vi "UI-电源尾反面标签2检测.vi"(8 "error in (no error)":errorcluster caption="错误输入（无错误）", 11 "名称或相对路径":string="Template Program") -> (0 "error in (no error) 2":errorcluster caption="错误输入（无错误）")   [LabVIEW 2017]
uses:
  Global System.vi
  <vilib>/Utility/xml.llb/Write to XML File(string).vi
  Picture/SaveButtom.ctl
panel:
  in  "获取图像":bool
  in  "ROI获取":bool
  in  "创建模板":bool
  in  "保存图像":bool
  out "添加的路径":path
  in  "刷新":bool
  in  "测试按钮":bool
  in  "保存按钮":bool
  in  "Main":enum32{"主参数", "模板匹配参数 ", "测试效果"}(tab)
  in  "UI电源尾反面标签2基础参数":T1={"IsNorImage"=TRUE, "Exposure Values"=100289, "ImagePath"=path "C:/Users/hedongpo/Desktop/514-hdp/Alignment Assemble System/Test Picture/B/3.bmp"} caption="参数界面" {"Exposure Values" scale=0.0..200000.0}
  in  "UI电源尾反面标签2参数":T3={"Rectangle"={"Left"=0, "Top"=0, "Right"=0, "Bottom"=0, "Rotation"=0.0}, "Algorithm "=2, "Parameters"={"Number of Matches Requested"=1, "Minimum Match Score"=800.0, "Angle Ranges"=[{"Start Angle"=-180.0, "End Angle"=180.0}]}, "Advanced Options "=[{"Item"=102, "Value"=10.0}, {"Item"=106, "Value"=300.0}, {"Item"=107, "Value"=0.0}, {"Item"=108, "Value"=6.0}, {"Item"=109, "Value"=1.0}, {"Item"=114, "Value"=25.0}, {"Item"=111, "Value"=20.0}, {"Item"=112, "Value"=10.0}, {"Item"=113, "Value"=20.0}, {"Item"=103, "Value"=1.0}, {"Item"=104, "Value"=20.0}, {"Item"=105, "Value"=0.0}, {"Item"=100, "Value"=5.0}], "模板路径"=path "", "Color Plane "=0} {"Color Plane" items=["Red", "Green", "Blue", "Hue", "Saturation", "Luminance", "Value", "Intensity"]; "Advanced Options"."Item" items=["LD Sampling - Minimum Constrast"=0, "LD Sampling - Enable Subpixel Accuracy"=1, "LD Sampling - Search Strategy"=2, "LD Sampling - Subpixel Iterations"=3, "LD Sampling - Subpixel Tolerance"=4, "LD Sampling - Initial Match List Length"=5, "LD Sampling - Match List Reduction Factor"=6, "LD Sampling - Initial Step Size"=7, "LD Sampling - Intermediate Angular Accuracy"=8, "-"=9, "Pyramid - Max Pyramid Level"=100, "Pyramid - Minimum Contrast"=102, "Pyramid - Enable Subpixel Accuracy"=103, "Pyramid - Subpixel Iterations"=104, "Pyramid - Subpixel Tolerance"=105, "Pyramid - Initial Match List Length"=106, "Pyramid - Match List Reduction Factor"=107, "Pyramid - Intermediate Angular Accuracy"=108, "Pyramid - Process Border Matches"=109, "Pyramid - Min Match Separation Distance"=111, "Pyramid - Min Match Separation Angle"=112, "Pyramid - Max Match Overlap"=113, "Pyramid - Max Cache in MB"=114, "Pyramid - Clear Cache"=115, "-"=116, "Enable Defect Map"=200]; "Algorithm" items=["All", "Low Discrepancy Sampling", "Grayscale Value Pyramid", "Gradients Pyramid"]; "Rectangle"."Rotation" format="%.2f"; "Rectangle"."Left" scale=0.0..1024.0; "Rectangle"."Right" scale=0.0..1024.0}
  out "结果":bool
  out "原始图像":T4(plugin-control)
  out "模板图片":T4(plugin-control)
  out "路径输出":path
  in  "Vision Paramter Save Buttom":T5
  out "system time":string
  in  "取消按钮":bool
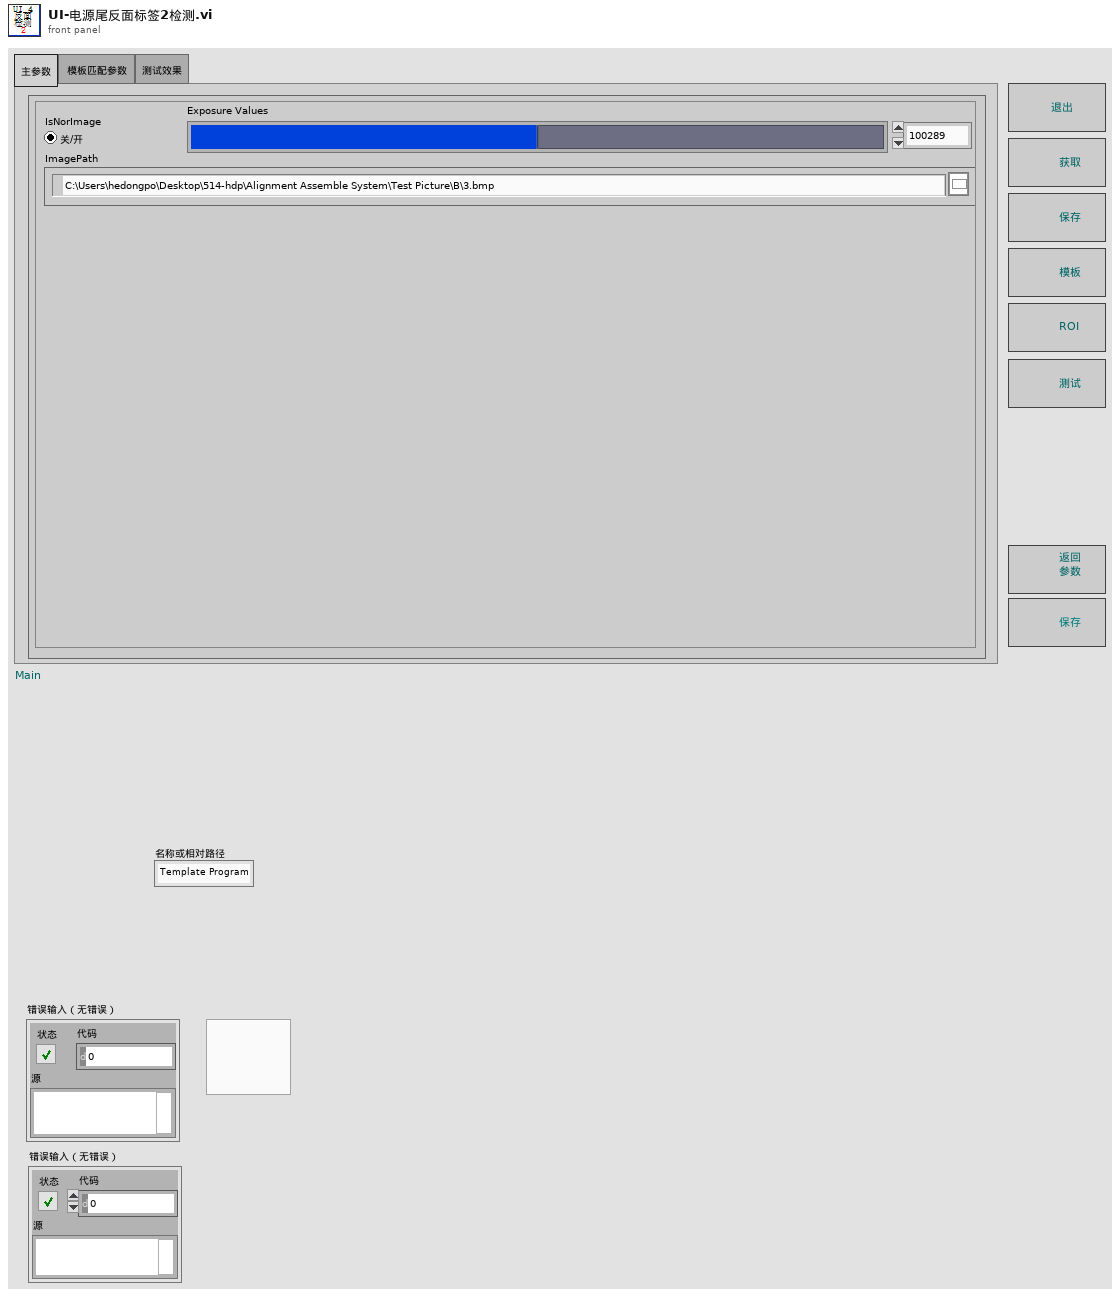
[diagram p1: front panel]
types:
  T1 = cluster{"IsNorImage":bool, "Exposure Values":u32, "ImagePath":path}
  T2 = typedef "IMAQ Rectangle" = cluster{"Left":i32, "Top":i32, "Right":i32, "Bottom":i32, "Rotation":dbl}
  T3 = cluster{"Rectangle":T2, "Algorithm ":i32, "Parameters":cluster{"Number of Matches Requested":i32, "Minimum Match Score":sgl, "Angle Ranges":cluster{"Start Angle":sgl, "End Angle":sgl}[]}, "Advanced Options ":cluster{"Item":u16, "Value":dbl}[], "模板路径":path, "Color Plane ":i32}
  T4 = typedef "IMAQ Image.ctl" = refnum<image>
  T5 = typedef "SaveButtom.ctl" = bool
  T6 = cluster{"index":i32, "this vi":refnum<vi>, "error out":errorcluster}
  T7 = cluster{"master data":string, "priority":u16, "secondary data":string[]}
  T8 = cluster{"case name":string[], "queue array":refnum<queue>[]}
  T9 = typedef "Image Type" = u32
  T10 = cluster{"Global Rectangle":i32[], "Contours":cluster{"Contour Type":u32, "ROI Type":u32, "Points":i32[]}[]}
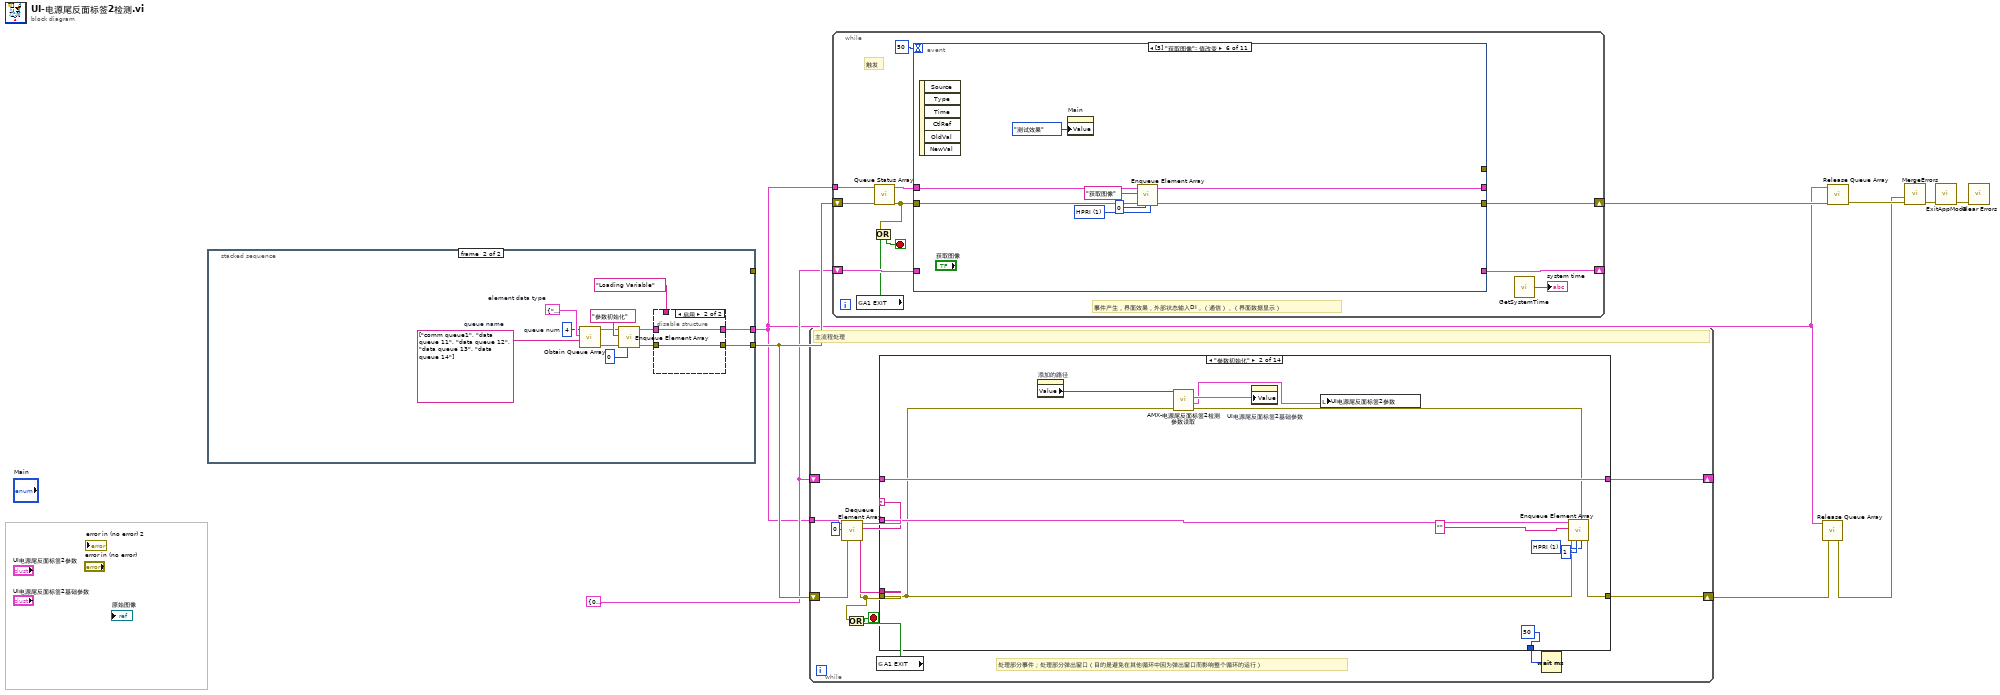
[diagram p0: block diagram]
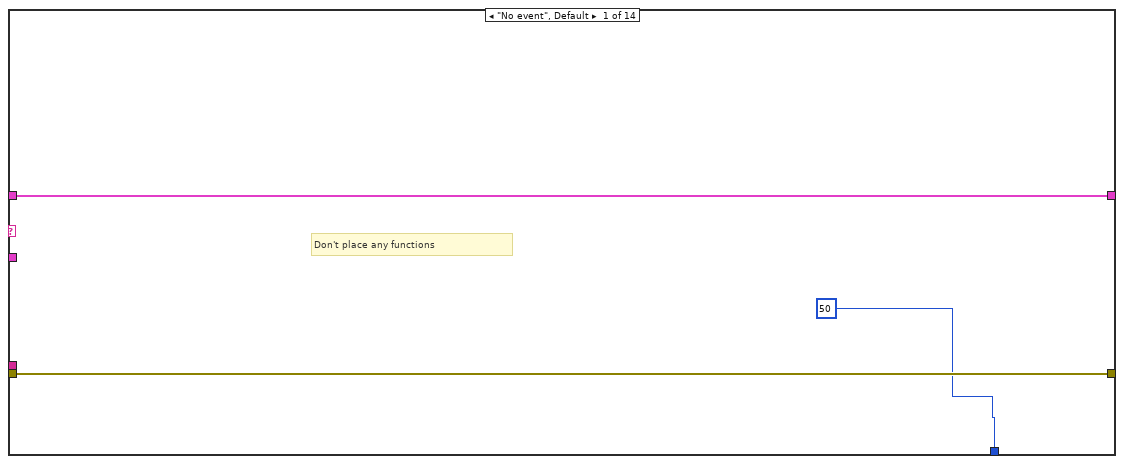
[diagram p2: hidden frame]
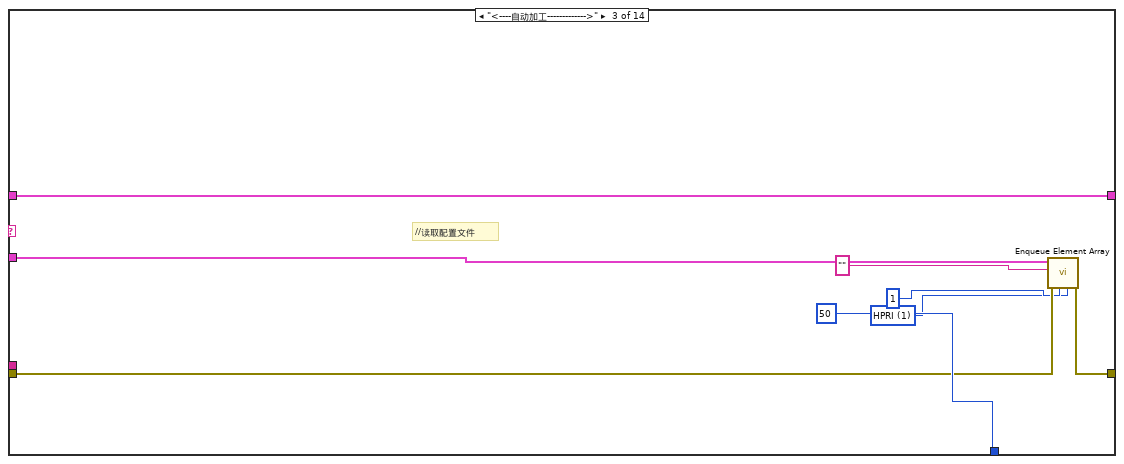
[diagram p3: hidden frame]
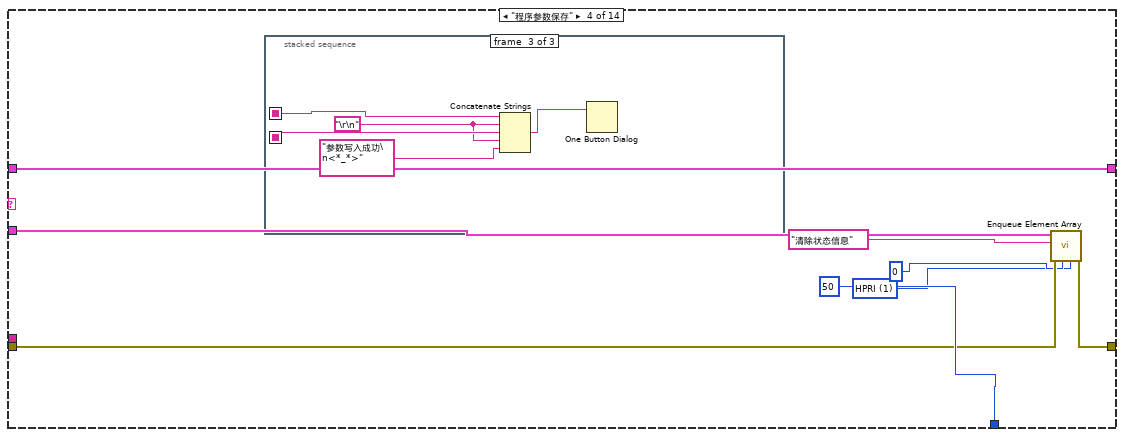
[diagram p4: hidden frame]
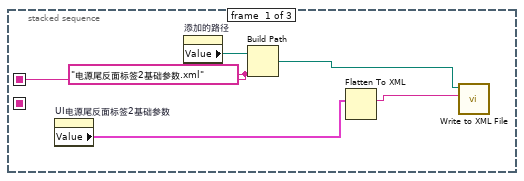
[diagram p5: hidden frame]
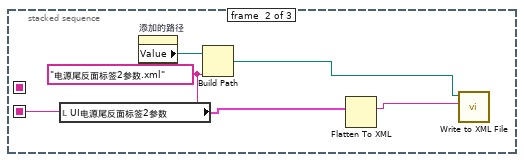
[diagram p6: hidden frame]
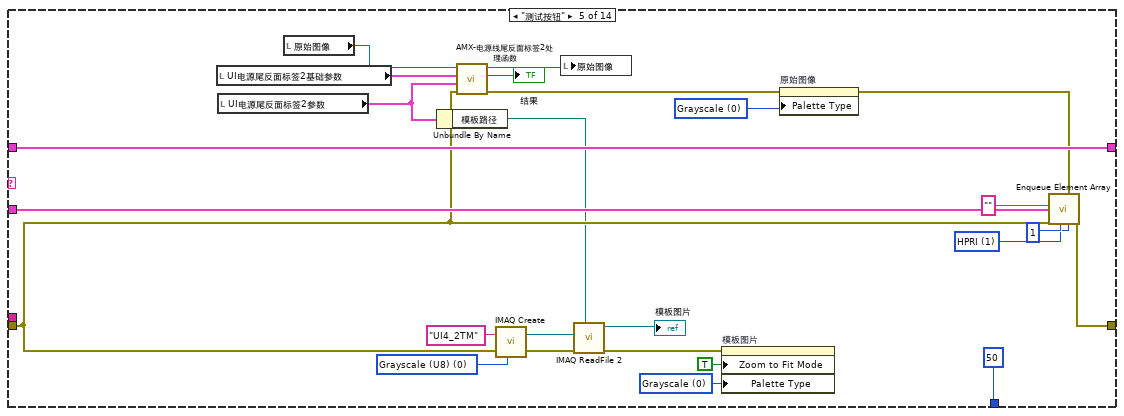
[diagram p7: hidden frame]
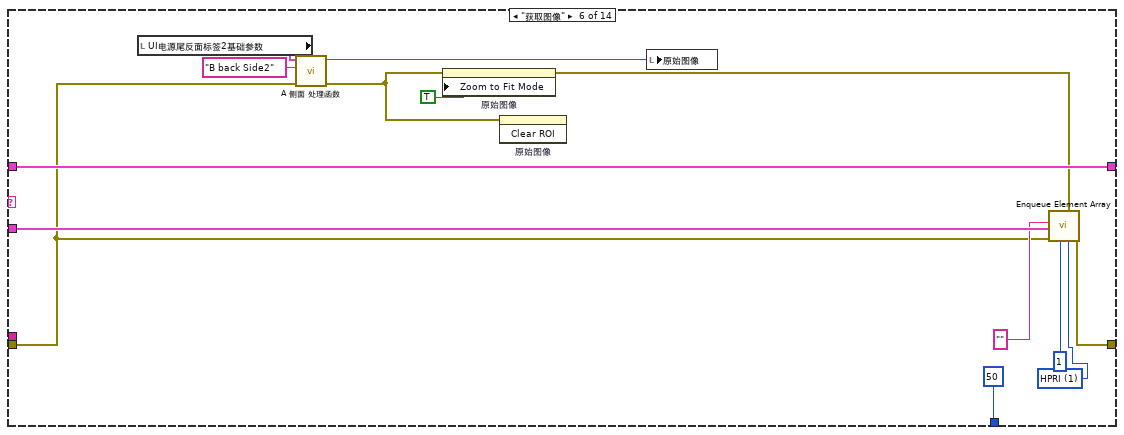
[diagram p8: hidden frame]
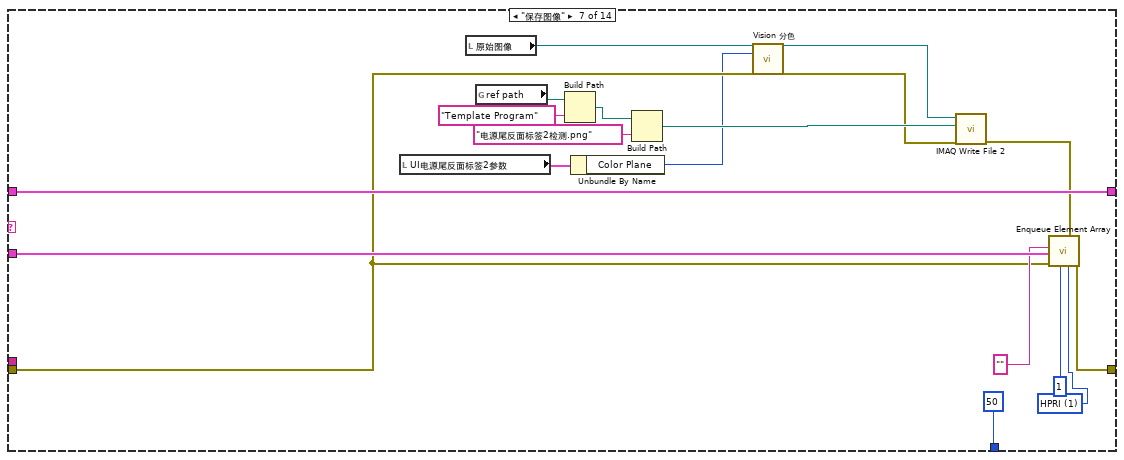
[diagram p9: hidden frame]
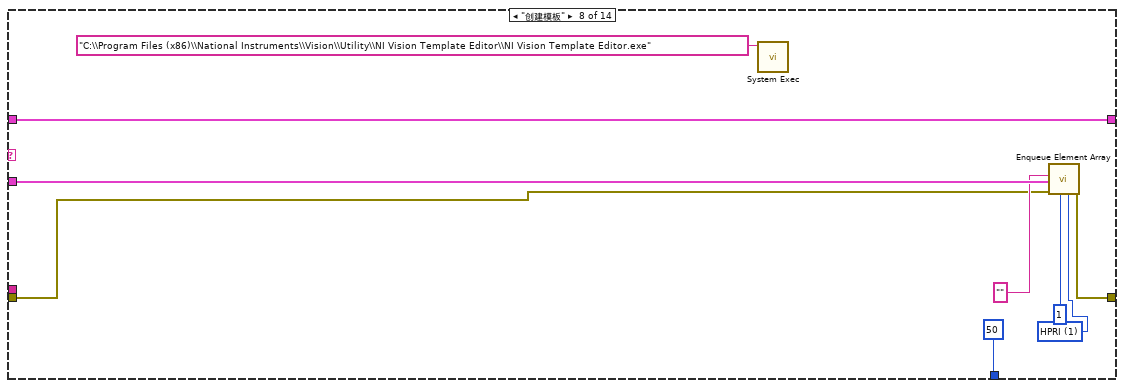
[diagram p10: hidden frame]
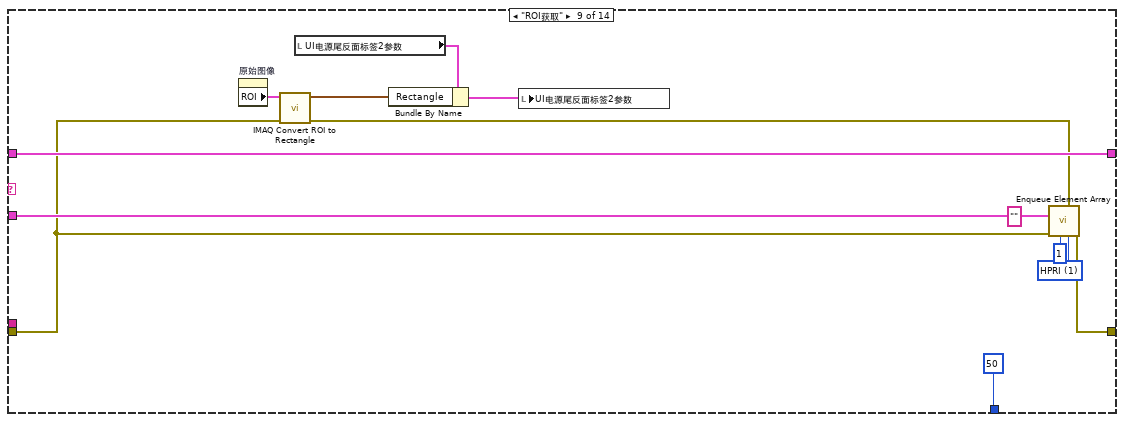
[diagram p11: hidden frame]
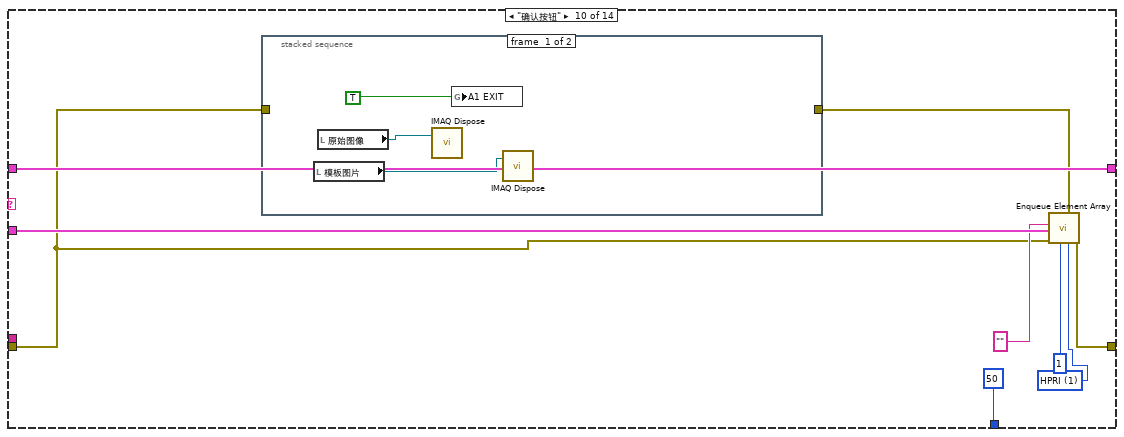
[diagram p12: hidden frame]
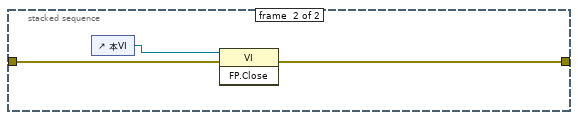
[diagram p13: hidden frame]
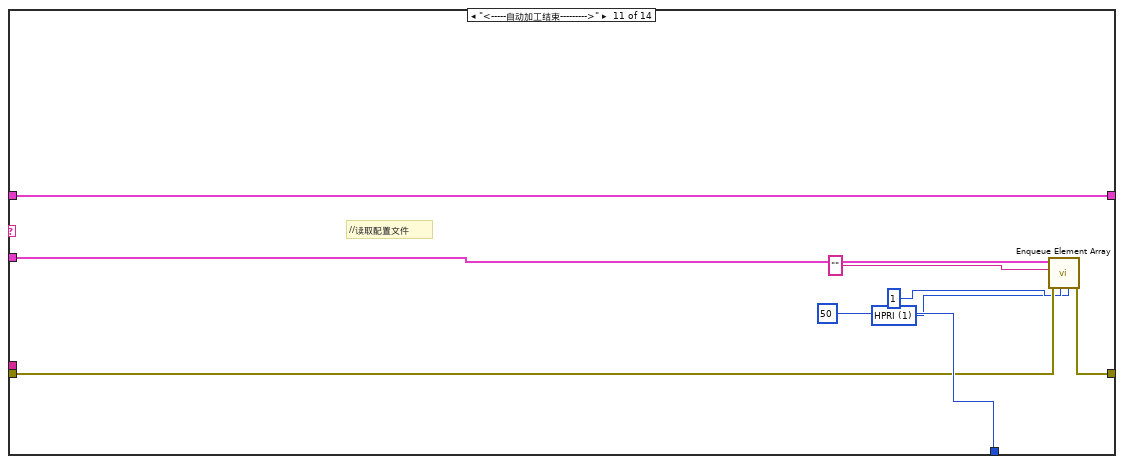
[diagram p14: hidden frame]
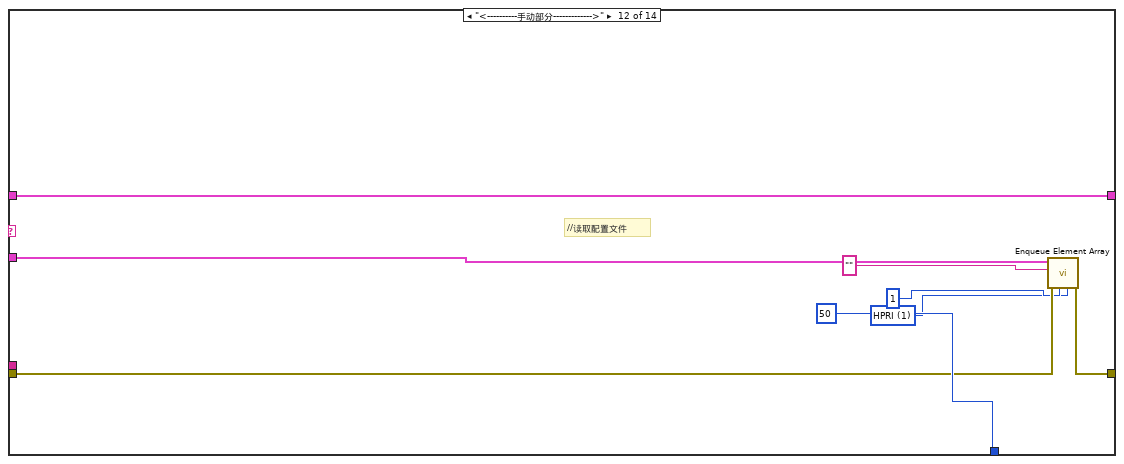
[diagram p15: hidden frame]
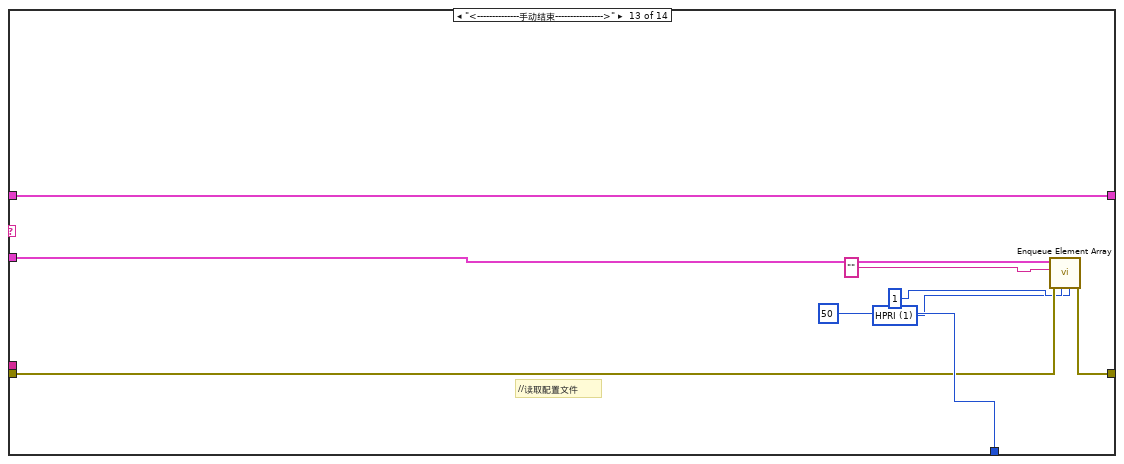
[diagram p16: hidden frame]
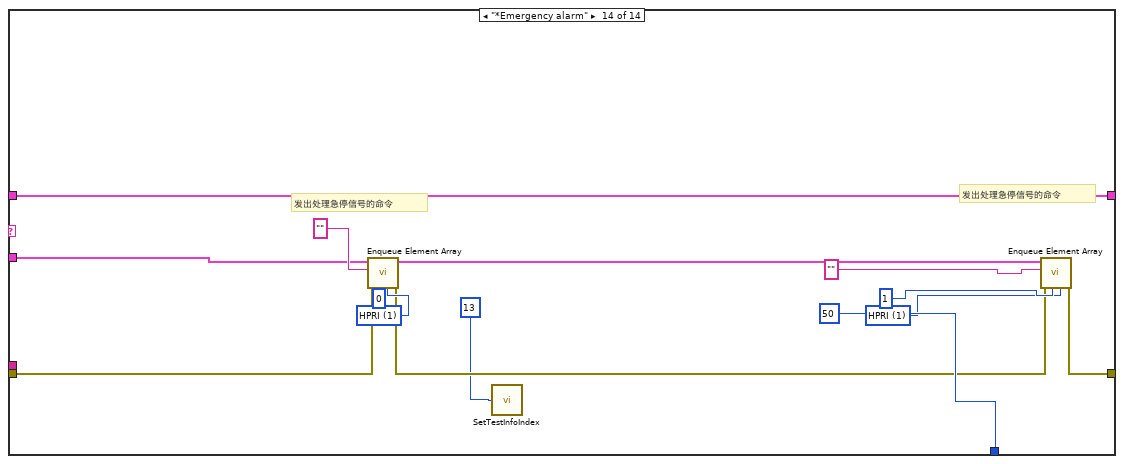
[diagram p17: hidden frame]
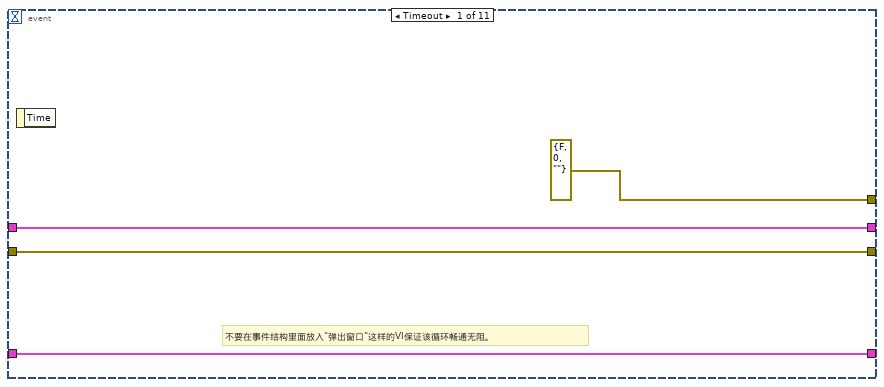
[diagram p18: hidden frame]
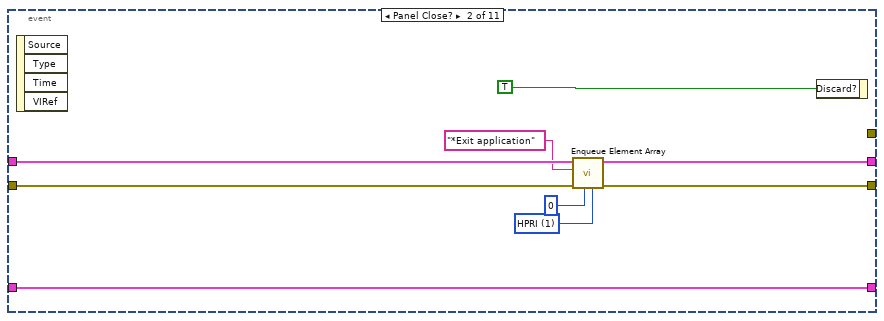
[diagram p19: hidden frame]
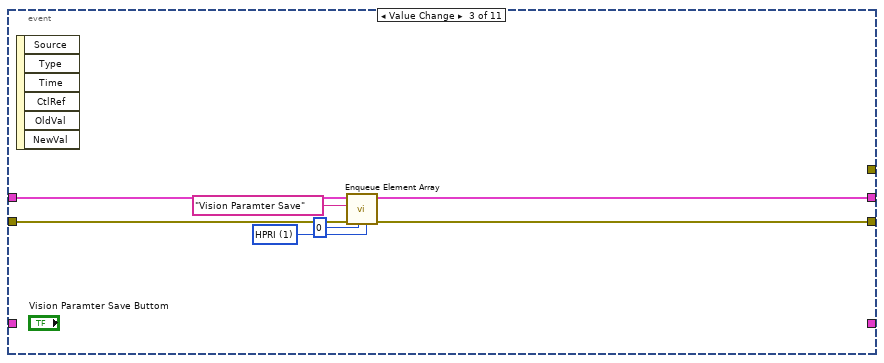
[diagram p20: hidden frame]
diagram:
  w4 = T6 {"index"=0, "this vi"=refnum, "error out"={"status"=FALSE, "code"=0, "source"=""}} ("parameter buffer")
  n1 = stacked-sequence {
    tunnel: [w15 _] -> _
    tunnel: [_ w19] -> w5
    tunnel: [_ w18] -> w1
    frame #0 {
      n2 = global read "Global System.vi" "ref path"() -> (w13:path)
      n3 = Build Path(base path=w13, name or relative path="Template Program" ("名称或相对路径")) -> (appended path=w11:path)
      n4 = property on="Main" class="TabCtl (严格)"("Value"=enum32{"主参数", "模板匹配参数 ", "测试效果"}."主参数" ("Main")) -> ()  [unwired: 2 in, 2 out]
      n5 = Build Path(base path=w11, name or relative path="名称或相对路径") -> (appended path=w17:path)
      "添加的路径" <- w17
      n6 = List Folder(path=w17) -> (path out=→"路径输出":path, error out=w15:errorcluster)  [unwired: 3 in, 2 out]
    }
    frame #1 {
      w27 = string[] ["comm queue1", "data queue 11", "data queue 12", "data queue 13", "data queue 14"]  # queue name
      w28 = 4  # queue num
      w29 = T7 {"master data"="", "priority"=0, "secondary data"=[]}  # element data type
      n7 = call "Obtain Queue Array.vi"("queue name"=w27, "element data type"=w29, "queue num"=w28) -> ("error out"=w23:errorcluster, "queue out"=w24:T8)  [unwired: 2 in, 1 out]
      n8 = call "Enqueue Element Array.vi"("queue index"=0, "error in"=w23, "master data"="参数初始化", "queue in"=w24) -> ("error out"=w22:errorcluster, "queue out"=w21:T8)  [unwired: 6 in]
      n9 = disable-structure shown="启用" {
        disable-tunnel: w22 -> [w35 w36]
        disable-tunnel: w21 -> [w34 w37]
        disable-tunnel: "Loading Variable" ("master data") -> [w33 _]
        disable-tunnel: [w31 w36] -> w19
        disable-tunnel: [w30 w37] -> w18
        frame Disabled {
          n10 = call "Enqueue Element Array.vi"("queue index"=12, "error in"=w35, "master data"=w33, "queue in"=w34) -> ("error out"=w31:errorcluster, "queue out"=w30:T8)  [unwired: 6 in]
        }
        frame Enabled {
        }
      }
    }
  }
  n11 = while {
    shift-right: [w50] -> w3
    shift-left: w5 -> [w41]
    shift-right: [w47] -> _
    shift-left: w4 -> [w48]
    tunnel: w1 -> [w43]
    stop <- w38 stop-if-true
    # "处理部分事件；处理部分弹出窗口（目的是避免在其他循环中因为弹出窗口而影响整个循环的运行）"
    # "主流程处理"
    n12 = call "Dequeue Element Array.vi"("queue in"=w43, "queue index"=0, "error in"=w41) -> ("queue out"=w46:T8, "master data"=w45:string, "secondary data"=w44:string[], "error out"=w40:errorcluster)  [unwired: 2 in, 1 out]
    n13 = global read "Global System.vi" "A1 EXIT"() -> (w39:bool)
    n14 = Or(x=w40, y=w39) -> (x .or. y?=w38:bool)
    n15 = case shown="\"参数初始化\"" w45 {
      tunnel: w46 -> [_ w64 w72 w74 w120 w134 w153 w162 w175 w184 w198 w206 w214 w220]
      tunnel: w40 -> [w52 w57 w68 w78 w113 w125 w139 w156 w168 w178 w194 w202 w210 w217]
      tunnel: [w52 w63 w71 w80 w119 w133 w152 w161 w174 w183 w197 w205 w213 w228] -> w50
      tunnel: [50 50 50 50 50 50 50 50 50 50 50 50 50 50] -> w49
      tunnel: w48 -> [w53 w59 w69 w75 w115 w129 w148 w157 w170 w179 w195 w203 w211 w226]
      tunnel: [w53 w59 w69 w75 w115 w129 w148 w157 w170 w179 w195 w203 w211 w226] -> w47
      tunnel: w44 -> [_ _ _ _ _ _ _ _ _ _ _ _ _ _]
      frame "No event", Default {
        # "Don't place any functions"
      }
      frame "参数初始化" {
        w60 = u16 1 items=["HPRI"=1, "LPRI"=0] ("priority")
        n16 = property on="添加的路径" class="Path"() -> ("Value"=w58:path)  [unwired: 2 in, 2 out]
        n17 = call "AMX-电源尾反面标签2检测参数读取.vi"("error in (no error)"=w57, "基路径"=w58) -> ("error out"=w54:errorcluster, "UI电源尾反面标签2参数"=w55:T3, "UI电源尾反面标签2基础参数"=w56:T1)  [unwired: 6 in]
        n18 = property on="UI电源尾反面标签2基础参数" class="Clust (严格)"("Value"=w56) -> ()  [unwired: 2 in, 2 out]
        n19 = local write "UI电源尾反面标签2参数"(w55) -> ()
        n20 = call "Enqueue Element Array.vi"("priority"=w60, "device error in"=w54, "queue index"=1, "error in"=w57, "master data"="" ("Element 1"), "queue in"=w64) -> ("error out"=w63:errorcluster)  [unwired: 4 in, 1 out]
      }
      frame "<----自动加工------------->" {
        w66 = u16 1 items=["HPRI"=1, "LPRI"=0] ("priority")
        # "//读取配置文件"
        n21 = call "Enqueue Element Array.vi"("priority"=w66, "queue index"=1, "error in"=w68, "master data"="" ("Element 1"), "queue in"=w72) -> ("error out"=w71:errorcluster)  [unwired: 5 in, 1 out]
      }
      frame "程序参数保存" {
        w76 = u16 1 items=["HPRI"=1, "LPRI"=0] ("priority")
        n22 = stacked-sequence {
          seq-local: [w82 _ _] -> [_ _ w95]
          seq-local: [_ w88 _] -> [_ _ w93]
          frame #0 {
            w82 = "电源尾反面标签2基础参数.xml" ("名称或相对路径")
            n23 = property on="UI电源尾反面标签2基础参数" class="Clust (严格)"() -> ("Value"=w85:T1)  [unwired: 2 in, 2 out]
            n24 = property on="添加的路径" class="Path"() -> ("Value"=w86:path)  [unwired: 2 in, 2 out]
            n25 = Build Path(base path=w86, name or relative path=w82) -> (appended path=w83:path)
            n26 = Flatten To XML(anything=w85) -> (xml string=w84:string)
            n27 = call-poly <vilib>:"Write to XML File.vi"("XML Input"=w84, "XML File Path"=w83) -> ()  [unwired: 7 in, 3 out]
          }
          frame #1 {
            w88 = "电源尾反面标签2参数.xml" ("名称或相对路径")
            n28 = local read "UI电源尾反面标签2参数"() -> (w87:T3)
            n29 = property on="添加的路径" class="Path"() -> ("Value"=w91:path)  [unwired: 2 in, 2 out]
            n30 = Build Path(base path=w91, name or relative path=w88) -> (appended path=w89:path)
            n31 = Flatten To XML(anything=w87) -> (xml string=w90:string)
            n32 = call-poly <vilib>:"Write to XML File.vi"("XML Input"=w90, "XML File Path"=w89) -> ()  [unwired: 7 in, 3 out]
          }
          frame #2 {
            w92 = "\r\n"
            n33 = Concatenate Strings(w95, w92, w93, w92, "参数写入成功\n<*_*>" ("消息")) -> (w94:string)
            n34 = One Button Dialog(message=w94) -> ()  [unwired: 1 in, 1 out]
          }
        }
        n35 = call "Enqueue Element Array.vi"("priority"=w76, "queue index"=0, "error in"=w78, "master data"="清除状态信息" ("Element 1"), "queue in"=w74) -> ("error out"=w80:errorcluster)  [unwired: 5 in, 1 out]
      }
      frame "测试按钮" {
        w100 = u32 0 items=["Grayscale", "Binary", "Gradient", "Rainbow", "Temperature", "User Defined", "Binary 16 Bit", "Gradient 16 Bit", "Rainbow 16 Bit", "Temperature 16 Bit", "User Defined 16 Bit"] ("Palette:Palette Type")
        w106 = T9 0 items=["Grayscale (U8)", "Grayscale (I16)", "Grayscale (SGL)", "Complex (CSG)", "RGB (U32)", "HSL (U32)", "RGB (U64)", "Grayscale (U16)"] ("Image Type")
        w108 = u32 0 items=["Grayscale", "Binary", "Gradient", "Rainbow", "Temperature", "User Defined", "Binary 16 Bit", "Gradient 16 Bit", "Rainbow 16 Bit", "Temperature 16 Bit", "User Defined 16 Bit"] ("Palette:Palette Type")
        w116 = u16 1 items=["HPRI"=1, "LPRI"=0] ("priority")
        n36 = local read "UI电源尾反面标签2基础参数"() -> (w114:T1)
        n37 = local read "UI电源尾反面标签2参数"() -> (w111:T3)
        n38 = local read "原始图像"() -> (w110:T4)
        n39 = Unbundle By Name(w111) -> ("模板路径"=w99:path)
        n40 = call "AMX-电源线尾反面标签2处理函数.vi"("error in (no error)"=w113, "UI电源线正面标签1参数"=w111, "电源线正面标签1基础参数"=w114, "Image in"=w110) -> ("error out"=w109:errorcluster, "j结果"=→"结果":bool, "Image out"=w112:T4)  [unwired: 4 in, 1 out]
        n41 = call "IMAQ Create"("Image Name"="UI4_2TM", "Image Type"=w106, "error in (no error)"=w113) -> ("New Image"=w105:T4, "error out"=w104:errorcluster)  [unwired: 2 in]
        n42 = local write "原始图像"(w112) -> ()
        n43 = call "IMAQ ReadFile 2"("File Path"=w99, "error in (no error)"=w104, "Image"=w105) -> ("error out"=w102:errorcluster, "Image Out"=→"模板图片":T4)  [unwired: 4 in, 3 out]
        n44 = property on="模板图片" class="ImageControl"(error in=w102, "Zoom to Fit Mode"=TRUE, "Palette Type"=w100) -> ()  [unwired: 1 in, 2 out]
        n45 = property on="原始图像" class="ImageControl"(error in=w109, "Palette Type"=w108) -> (error out=w97:errorcluster)  [unwired: 1 in, 1 out]
        n46 = call "Enqueue Element Array.vi"("priority"=w116, "device error in"=w97, "queue index"=1, "error in"=w113, "master data"="" ("Element 1"), "queue in"=w120) -> ("error out"=w119:errorcluster)  [unwired: 4 in, 1 out]
      }
      frame "获取图像" {
        w130 = u16 1 items=["HPRI"=1, "LPRI"=0] ("priority")
        n47 = local read "UI电源尾反面标签2基础参数"() -> (w127:T1)
        n48 = call "A 侧面 处理函数.vi"("error in (no error)"=w125, "Image Name"="B back Side2", "ParamsUI"=w127) -> ("error out"=w122:errorcluster, "Image out"=w126:T4)  [unwired: 5 in, 2 out]
        n49 = property on="原始图像" class="ImageControl"(error in=w122, "Zoom to Fit Mode"=TRUE) -> (error out=w123:errorcluster)  [unwired: 1 in, 1 out]
        n50 = invoke on="原始图像" class="ImageControl" method="Clear ROI"(error in=w122) -> ()  [unwired: 2 in, 3 out]
        n51 = local write "原始图像"(w126) -> ()
        n52 = call "Enqueue Element Array.vi"("priority"=w130, "device error in"=w123, "queue index"=1, "error in"=w125, "master data"="" ("Element 1"), "queue in"=w134) -> ("error out"=w133:errorcluster)  [unwired: 4 in, 1 out]
      }
      frame "保存图像" {
        w149 = u16 1 items=["HPRI"=1, "LPRI"=0] ("priority")
        n53 = local read "UI电源尾反面标签2参数"() -> (w137:T3)
        n54 = local read "原始图像"() -> (w141:T4)
        n55 = global read "Global System.vi" "ref path"() -> (w147:path)
        n56 = Build Path(base path=w147, name or relative path="Template Program" ("名称或相对路径")) -> (appended path=w145:path)
        n57 = Unbundle By Name(w137) -> ("Color Plane"=w136:i32)
        n58 = Build Path(base path=w145, name or relative path="电源尾反面标签2检测.png" ("名称或相对路径")) -> (appended path=w143:path)
        n59 = call "Vision 分色"("Image In"=w141, "Color Plane (Color Plane Extraction 1)"=w136, "error in"=w139) -> ("Image Out"=w140:T4, "error out"=w138:errorcluster)  [unwired: 23 in]
        n60 = call-poly "IMAQ Write File 2"("error in (no error)"=w138, "File Path"=w143, "Image"=w140) -> ("error out"=w142:errorcluster)  [unwired: 7 in, 1 out]
        n61 = call "Enqueue Element Array.vi"("priority"=w149, "device error in"=w142, "queue index"=1, "error in"=w139, "master data"="" ("Element 1"), "queue in"=w153) -> ("error out"=w152:errorcluster)  [unwired: 4 in, 1 out]
      }
      frame "创建模板" {
        w158 = u16 1 items=["HPRI"=1, "LPRI"=0] ("priority")
        n62 = call <vilib>:"System Exec.vi"("command line"="C:\\Program Files (x86)\\National Instruments\\Vision\\Utility\\NI Vision Template Editor\\NI Vision Template Editor.exe") -> ()  [unwired: 7 in, 4 out]
        n63 = call "Enqueue Element Array.vi"("priority"=w158, "queue index"=1, "error in"=w156, "master data"="" ("Element 1"), "queue in"=w162) -> ("error out"=w161:errorcluster)  [unwired: 5 in, 1 out]
      }
      frame "ROI获取" {
        w171 = u16 1 items=["HPRI"=1, "LPRI"=0] ("priority")
        n64 = property on="原始图像" class="ImageControl"() -> ("ROI"=w169:T10)  [unwired: 2 in, 2 out]
        n65 = call "IMAQ Convert ROI to Rectangle"("error in (no error)"=w168, "ROI Descriptor"=w169) -> ("error out"=w164:errorcluster, "Rectangle"=w166:T2)  [unwired: 7 in]
        n66 = local read "UI电源尾反面标签2参数"() -> (w167:T3)
        n67 = Bundle By Name(cluster=w167, "Rectangle"=w166) -> (w165:T3)
        n68 = local write "UI电源尾反面标签2参数"(w165) -> ()
        n69 = call "Enqueue Element Array.vi"("priority"=w171, "device error in"=w164, "queue index"=1, "error in"=w168, "master data"="" ("Element 1"), "queue in"=w175) -> ("error out"=w174:errorcluster)  [unwired: 4 in, 1 out]
      }
      frame "确认按钮" {
        w180 = u16 1 items=["HPRI"=1, "LPRI"=0] ("priority")
        n70 = stacked-sequence {
          tunnel: w178 -> [_ w190]
          tunnel: [_ w189] -> w177
          frame #0 {
            n71 = local read "模板图片"() -> (w186:T4)
            n72 = local read "原始图像"() -> (w187:T4)
            n73 = call "IMAQ Dispose"("Image"=w187) -> ()  [unwired: 5 in, 1 out]
            n74 = global write "Global System.vi" "A1 EXIT"(TRUE ("EXIT")) -> ()
            n75 = call "IMAQ Dispose"("Image"=w186) -> ()  [unwired: 5 in, 1 out]
          }
          frame #1 {
            n76 = control-ref of="本VI"() -> (w191:refnum<vi>)
            n77 = invoke class="VI" method="FP.Close"(reference=w191, error in=w190) -> (error out=w189:errorcluster)  [unwired: 1 in, 2 out]
          }
        }
        n78 = call "Enqueue Element Array.vi"("priority"=w180, "device error in"=w177, "queue index"=1, "error in"=w178, "master data"="" ("Element 1"), "queue in"=w184) -> ("error out"=w183:errorcluster)  [unwired: 4 in, 1 out]
      }
      frame "<-----自动加工结束--------->" {
        w192 = u16 1 items=["HPRI"=1, "LPRI"=0] ("priority")
        # "//读取配置文件"
        n79 = call "Enqueue Element Array.vi"("priority"=w192, "queue index"=1, "error in"=w194, "master data"="" ("Element 1"), "queue in"=w198) -> ("error out"=w197:errorcluster)  [unwired: 5 in, 1 out]
      }
      frame "<----------手动部分------------->" {
        w200 = u16 1 items=["HPRI"=1, "LPRI"=0] ("priority")
        # "//读取配置文件"
        n80 = call "Enqueue Element Array.vi"("priority"=w200, "queue index"=1, "error in"=w202, "master data"="" ("Element 1"), "queue in"=w206) -> ("error out"=w205:errorcluster)  [unwired: 5 in, 1 out]
      }
      frame "<--------------手动结束---------------->" {
        w208 = u16 1 items=["HPRI"=1, "LPRI"=0] ("priority")
        # "//读取配置文件"
        n81 = call "Enqueue Element Array.vi"("priority"=w208, "queue index"=1, "error in"=w210, "master data"="" ("Element 1"), "queue in"=w214) -> ("error out"=w213:errorcluster)  [unwired: 5 in, 1 out]
      }
      frame "*Emergency alarm" {
        w223 = u16 1 items=["HPRI"=1, "LPRI"=0] ("priority")
        w224 = u16 1 items=["HPRI"=1, "LPRI"=0] ("priority")
        # "发出处理急停信号的命令"
        # "发出处理急停信号的命令"
        n82 = call "Enqueue Element Array.vi"("priority"=w223, "queue index"=0, "error in"=w217, "master data"="" ("Element 1"), "queue in"=w220) -> ("error out"=w218:errorcluster, "queue out"=w219:T8)  [unwired: 5 in]
        n83 = call "SetTestInfoIndex.vi"("test info index"=13) -> ()
        n84 = call "Enqueue Element Array.vi"("priority"=w224, "queue index"=1, "error in"=w218, "master data"="" ("Element 1"), "queue in"=w219) -> ("error out"=w228:errorcluster)  [unwired: 5 in, 1 out]
      }
    }
    n85 = Wait (ms)(milliseconds to wait=w49) -> ()  [unwired: 1 out]
  }
  n86 = while {
    shift-right: [w233] -> w6
    shift-left: w5 -> [w237]
    shift-right: [w235] -> _
    shift-left: w4 -> [w236]
    tunnel: w1 -> [w239]
    stop <- w230 stop-if-true
    # "触发"
    # "事件产生，界面效果，外部状态输入DI，（通信），（界面数据显示）"
    n87 = global read "Global System.vi" "A1 EXIT"() -> (w231:bool)
    n88 = call "Queue Status Array.vi"("error in (no error)"=w237, "queue in"=w239) -> ("error out"=w232:errorcluster, "queue out"=w234:T8)  [unwired: 4 in]
    n89 = Or(x=w232, y=w231) -> (x .or. y?=w230:bool)
    n90 = event shown="[5] \"获取图像\": 值改变" {
      selector: _ -> [_ _ _ _ _ _ _ _ _ _ _]
      dyn-events: _ -> [_ _ _ _ _ _ _ _ _ _ _]
      timeout: 50 -> [_ _ _ _ _ _ _ _ _ _ _]
      tunnel: w236 -> [w244 w252 _ _ _ _ _ _ _ _ _]
      tunnel: [w244 w252 _ _ _ _ _ _ _ _ _] -> w235
      tunnel: [errorcluster {"status"=FALSE, "code"=0, "source"=""} ("error out") _ _ _ _ _ _ _ _ _ _] -> _
      tunnel: w234 -> [w242 w251 w257 w264 w271 w279 w286 w293 w301 w309 w317]
      tunnel: w232 -> [w241 w250 w256 w263 w270 w278 w285 w292 w300 w308 w316]
      tunnel: [w241 w249 w254 w261 w268 w276 w283 w290 w298 w306 w314] -> w233
      tunnel: [w242 w248 w255 w262 w269 w277 w284 w291 w299 w307 w315] -> _
      event Timeout {
        # "不要在事件结构里面放入\"弹出窗口\"这样的VI保证该循环畅通无阻。"
        n91 = event-data() -> ()  [unwired: 1 in, 1 out]
      }
      event Panel Close? {
        w246 = u16 1 items=["HPRI"=1, "LPRI"=0] ("priority")
        n92 = event-data() -> ()  [unwired: 1 in, 4 out]
        n93 = call "Enqueue Element Array.vi"("priority"=w246, "queue index"=0, "error in"=w250, "master data"="*Exit application", "queue in"=w251) -> ("error out"=w249:errorcluster, "queue out"=w248:T8)  [unwired: 5 in]
        n94 = event-data("Discard?"=TRUE) -> ()  [unwired: 1 in, 1 out]
      }
      event Value Change {
        w259 = u16 1 items=["HPRI"=1, "LPRI"=0] ("priority")
        n95 = event-data() -> ()  [unwired: 1 in, 6 out]
        n96 = call "Enqueue Element Array.vi"("priority"=w259, "queue index"=0, "error in"=w256, "master data"="Vision Paramter Save", "queue in"=w257) -> ("error out"=w254:errorcluster, "queue out"=w255:T8)  [unwired: 5 in]
      }
      event "取消按钮": Value Change {
        w266 = u16 1 items=["HPRI"=1, "LPRI"=0] ("priority")
        n97 = event-data() -> ()  [unwired: 1 in, 6 out]
        n98 = call "Enqueue Element Array.vi"("priority"=w266, "queue index"=0, "error in"=w263, "master data"="确认按钮", "queue in"=w264) -> ("error out"=w261:errorcluster, "queue out"=w262:T8)  [unwired: 5 in]
      }
      event "保存按钮": Value Change {
        w273 = u16 1 items=["HPRI"=1, "LPRI"=0] ("priority")
        n99 = event-data() -> ()  [unwired: 1 in, 6 out]
        n100 = call "Enqueue Element Array.vi"("priority"=w273, "queue index"=0, "error in"=w270, "master data"="程序参数保存", "queue in"=w271) -> ("error out"=w268:errorcluster, "queue out"=w269:T8)  [unwired: 5 in]
      }
      event "获取图像": Value Change {
        w281 = u16 1 items=["HPRI"=1, "LPRI"=0] ("priority")
        n101 = event-data() -> ()  [unwired: 1 in, 6 out]
        n102 = property on="Main" class="TabCtl (严格)"("Value"=enum32{"主参数", "模板匹配参数 ", "测试效果"}."测试效果" ("Main")) -> ()  [unwired: 2 in, 2 out]
        n103 = call "Enqueue Element Array.vi"("priority"=w281, "queue index"=0, "error in"=w278, "master data"="获取图像", "queue in"=w279) -> ("error out"=w276:errorcluster, "queue out"=w277:T8)  [unwired: 5 in]
      }
      event "保存图像": Value Change {
        w288 = u16 1 items=["HPRI"=1, "LPRI"=0] ("priority")
        n104 = event-data() -> ()  [unwired: 1 in, 6 out]
        n105 = call "Enqueue Element Array.vi"("priority"=w288, "queue index"=0, "error in"=w285, "master data"="保存图像", "queue in"=w286) -> ("error out"=w283:errorcluster, "queue out"=w284:T8)  [unwired: 5 in]
      }
      event "创建模板": Value Change {
        w295 = u16 1 items=["HPRI"=1, "LPRI"=0] ("priority")
        n106 = event-data() -> ()  [unwired: 1 in, 6 out]
        n107 = call "Enqueue Element Array.vi"("priority"=w295, "queue index"=0, "error in"=w292, "master data"="创建模板", "queue in"=w293) -> ("error out"=w290:errorcluster, "queue out"=w291:T8)  [unwired: 5 in]
      }
      event "ROI获取": Value Change {
        w303 = u16 1 items=["HPRI"=1, "LPRI"=0] ("priority")
        n108 = event-data() -> ()  [unwired: 1 in, 6 out]
        n109 = property on="Main" class="TabCtl (严格)"("Value"=enum32{"主参数", "模板匹配参数 ", "测试效果"}."模板匹配参数 " ("Main")) -> ()  [unwired: 2 in, 2 out]
        n110 = call "Enqueue Element Array.vi"("priority"=w303, "queue index"=0, "error in"=w300, "master data"="ROI获取", "queue in"=w301) -> ("error out"=w298:errorcluster, "queue out"=w299:T8)  [unwired: 5 in]
      }
      event "测试按钮": Value Change {
        w311 = u16 1 items=["HPRI"=1, "LPRI"=0] ("priority")
        n111 = event-data() -> ()  [unwired: 1 in, 6 out]
        n112 = property on="Main" class="TabCtl (严格)"("Value"=enum32{"主参数", "模板匹配参数 ", "测试效果"}."测试效果" ("Main")) -> ()  [unwired: 2 in, 2 out]
        n113 = call "Enqueue Element Array.vi"("priority"=w311, "queue index"=0, "error in"=w308, "master data"="测试按钮", "queue in"=w309) -> ("error out"=w306:errorcluster, "queue out"=w307:T8)  [unwired: 5 in]
      }
      event "刷新": Value Change {
        n114 = event-data() -> ()  [unwired: 1 in, 6 out]
        n115 = disable-structure shown="禁用" {
          disable-tunnel: w317 -> [w321 _]
          disable-tunnel: w316 -> [w320 _]
          disable-tunnel: [w319 _] -> w315
          disable-tunnel: [w318 _] -> w314
          frame Disabled {
            w323 = u16 1 items=["HPRI"=1, "LPRI"=0] ("priority")
            # "刷新"
            n116 = call "Enqueue Element Array.vi"("priority"=w323, "queue index"=0, "error in"=w320, "master data"="刷新", "queue in"=w321) -> ("error out"=w318:errorcluster, "queue out"=w319:T8)  [unwired: 5 in]
          }
          frame Enabled {
          }
        }
        n117 = property on="Main" class="TabCtl (严格)"("Value"=enum32{"主参数", "模板匹配参数 ", "测试效果"}."模板匹配参数 " ("Main")) -> ()  [unwired: 2 in, 2 out]
      }
    }
    n118 = call "GetSystemTime.vi"() -> ("date/time string"=→"system time":string)  [unwired: 7 in]
  }
  n119 = call "Release Queue Array.vi"("error in"=w3, "queue in"=w1) -> ("error out"=w2:errorcluster)  [unwired: 2 in, 3 out]
  n120 = call "Release Queue Array.vi"("error in"=w6, "queue in"=w1) -> ("error out"=w9:errorcluster)  [unwired: 2 in, 3 out]
  n121 = call "MergeErrors.vi"("error in 3 (no error)"=w2, "error in 4 (no error)"=w9) -> ("error out"=w8:errorcluster)  [unwired: 6 in]
  n122 = call "ExitAppMode.vi"("error in (no error)"=w8) -> ("error out"=w7:errorcluster)  [unwired: 10 in]
  n123 = call <vilib>:"Clear Errors.vi"("error in (no error)"=w7) -> ()  [unwired: 5 in, 2 out]
